vi "AWGUpdateWaveformViewer.vi"(10 "Wave Form preview ref":refnum<vi>, 11 "Item Names":dbl[][](array[numeric])) -> ()   [LabVIEW 2019]
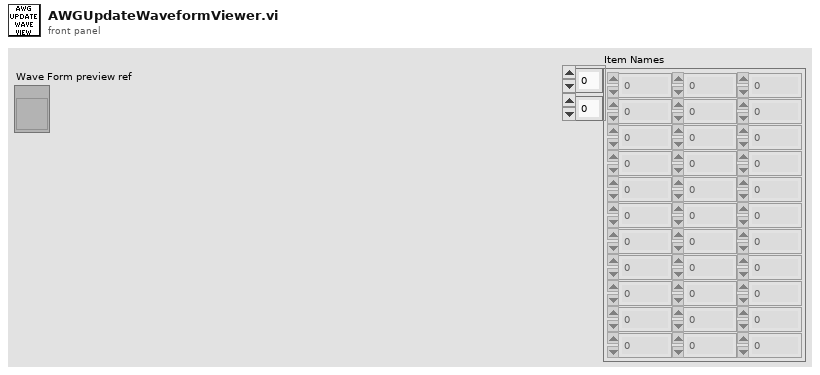
[diagram p1: front panel]
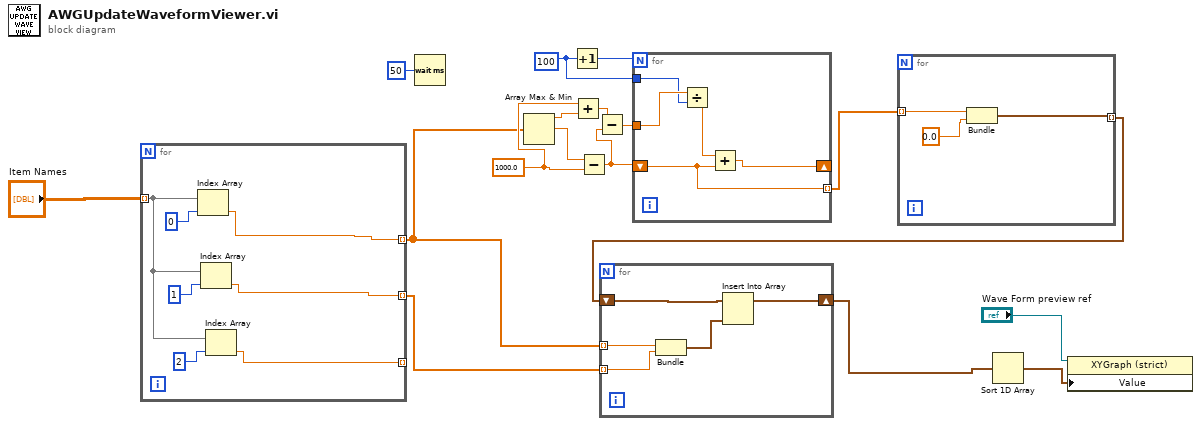
[diagram p0: block diagram]
diagram:
  w12 = 1000.0 ("y")
  w5 = 100
  n1 = for {
    tunnel: "Item Names" -> [w21] mode=indexing
    tunnel: [w18] -> _ mode=indexing
    tunnel: [w19] -> w7 mode=indexing
    tunnel: [w20] -> w9 mode=indexing
    n2 = Index Array(array=w21, index=0) -> (element=w20:dbl)
    n3 = Index Array(array=w21, index=1) -> (element=w19:dbl)
    n4 = Index Array(array=w21, index=2) -> (element=w18:dbl)
  }
  n5 = Wait (ms)(milliseconds to wait=u32 50) -> ()  [unwired: 1 out]
  n6 = Array Max & Min(array=w9) -> (max value=w14:dbl, min value=w15:dbl)  [unwired: 2 out]
  n7 = Increment(x=w5) -> (x+1=w6:i32)
  n8 = Add(x=w12, y=w14) -> (x+y=w13:dbl)
  n9 = Subtract(x=w15, y=w12) -> (x-y=w11:dbl)
  n10 = Subtract(x=w13, y=w11) -> (x-y=w16:dbl)
  n11 = for {
    N: w6 -> [_]
    tunnel: w16 -> [w29]
    shift-right: [w28] -> _
    shift-left: w11 -> [w26]
    tunnel: [w26] -> w10 mode=indexing
    tunnel: w5 -> [w25]
    n12 = Divide(x=w29, y=w25) -> (x/y=w27:dbl)
    n13 = Add(x=w27, y=w26) -> (x+y=w28:dbl)
  }
  n14 = for {
    tunnel: w10 -> [w32] mode=indexing
    tunnel: [w30] -> w8 mode=indexing
    n15 = Bundle(w32, 0.0) -> (w30:cluster{dbl, dbl})  [unwired: 1 in]
  }
  n16 = for {
    tunnel: w9 -> [w35] mode=indexing
    tunnel: w7 -> [w34] mode=indexing
    shift-right: [w37] -> w4
    shift-left: w8 -> [w36]
    n17 = Bundle(w35, w34) -> (w33:cluster{dbl, dbl})  [unwired: 1 in]
    n18 = Insert Into Array(array=w36, new element=w33) -> (w37:cluster{dbl, dbl}[])  [unwired: 1 in]
  }
  n19 = Sort 1D Array(array=w4) -> (sorted array=w3:cluster{dbl, dbl}[])
  n20 = property class="XYGraph (strict)"(reference="Wave Form preview ref", "Value"=w3) -> ()  [unwired: 1 in, 2 out]
